vi "Prime number loop.vi"(10 "Numeric Control":dbl) -> (2 "Not Prime":bool)   [LabVIEW 2012]
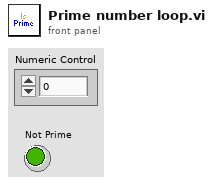
[diagram p1: front panel]
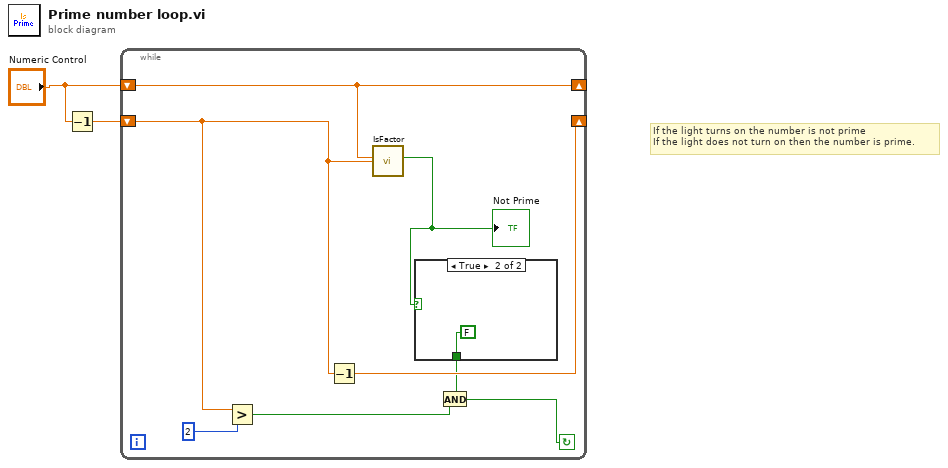
[diagram p0: block diagram]
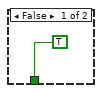
[diagram p2: hidden frame]
diagram:
  # "If the light turns on the number is not prime\nIf the light does not turn on then the number is prime."
  n1 = Decrement(x="Numeric Control") -> (x-1=w1:dbl)
  n2 = while {
    shift-right: [w5] -> _
    shift-left: "Numeric Control" -> [w5]
    shift-right: [w10] -> _
    shift-left: w1 -> [w4]
    stop <- w7 continue-if-true
    n3 = Greater?(x=w4, y=2) -> (0:w8:bool)
    n4 = Decrement(x=w4) -> (x-1=w10:dbl)
    n5 = call "IsFactor.vi"("Numeric Control 2"=w4, "Numeric Control"=w5) -> ("Boolean"=w3:bool)  [unwired: 9 in]
    "Not Prime" <- w3
    n6 = case shown="True" w3 {
      tunnel: [TRUE FALSE] -> w6
      frame False {
      }
      frame True {
      }
    }
    n7 = And(x=w6, y=w8) -> (x .and. y?=w7:bool)
  }
